vi "WallDistance.vi"(8 "Nominal Angle":dbl=90.0 format="%#_13g", 11 "Points":cluster{"X":sgl, "Y":sgl}[](array[cluster]) {"Y" format="%.2f"; "X" format="%.2f"}) -> (0 "Angle (deg)":dbl, 1 "y-Mean":sgl, 2 "x-Mean":sgl, 3 "Valid":bool, 4 "Segment":T1 {"Point 2"."Y" format="%.2f"; "Point 2"."X" format="%.2f"; "Point 1"."Y" format="%.2f"; "Point 1"."X" format="%.2f"}, 5 "Graph":cluster{sgl[], sgl[]})   [LabVIEW 2015]
uses:
  <vilib>/vision/NI_Vision_Development_Module.lvlib
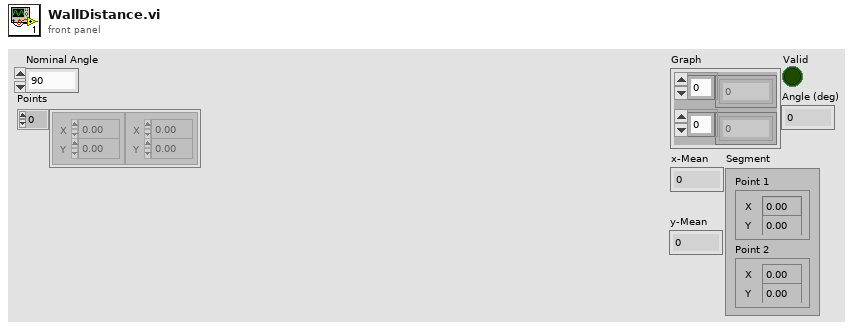
[diagram p1: front panel]
types:
  T1 = cluster{"Point 1":cluster{"X":sgl, "Y":sgl}, "Point 2":cluster{"X":sgl, "Y":sgl}}
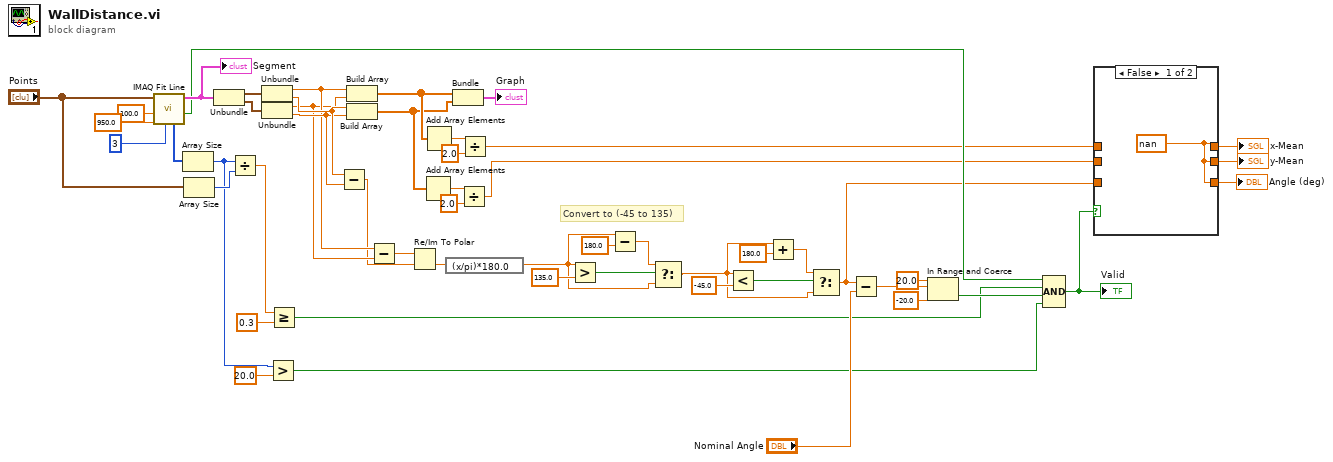
[diagram p0: block diagram]
diagram:
  # "Convert to (-45 to 135)"
  n1 = call "IMAQ Fit Line"("Maximum Iterations"=3, "Pixel Radius"=sgl 100.0, "Minimum Score"=sgl 950.0, "Points"="Points") -> ("Valid Fit?"=w16:bool, "Line Segment"=w21:T1, "Indexes of Points Used"=w23:i32[])  [unwired: 2 in, 3 out]
  "Segment" <- w21
  n2 = Array Size(array=w23) -> (size(s)=w10:i32)
  n3 = Array Size(array="Points") -> (size(s)=w22:i32)
  n4 = Unbundle(w21) -> ("Point 1"=w52:cluster{"X":sgl, "Y":sgl}, "Point 2"=w51:cluster{"X":sgl, "Y":sgl})
  n5 = Divide(x=w10, y=w22) -> (x/y=w15:dbl)
  n6 = Unbundle(w52) -> ("X"=w41:sgl, "Y"=w43:sgl)
  n7 = Unbundle(w51) -> ("X"=w40:sgl, "Y"=w42:sgl)
  n8 = Greater?(x=w10, y=20.0) -> (0:w9:bool)
  n9 = Greater Or Equal?(x=w15, y=0.3) -> (x >= y?=w13:bool)
  n10 = Subtract(x=w43, y=w42) -> (x-y=w38:sgl)
  n11 = Build Array(w41, w40) -> (w49:sgl[])
  n12 = Build Array(w43, w42) -> (w44:sgl[])
  n13 = Subtract(x=w41, y=w40) -> (x-y=w39:sgl)
  n14 = Re/Im To Polar(2:w38, 3:w39) -> (0:w28:sgl)  [unwired: 1 out]
  n15 = Add Array Elements(numeric array=w44) -> (sum=w45:sgl)
  n16 = Add Array Elements(numeric array=w49) -> (sum=w48:sgl)
  n17 = expression code="(x/pi)*180.0" ("radians to degrees")(w28) -> (w27:sgl)
  n18 = Bundle(w49, w44) -> (→"Graph":cluster{sgl[], sgl[]})  [unwired: 1 in]
  n19 = Divide(x=w45, y=sgl 2.0) -> (x/y=w5:sgl)
  n20 = Divide(x=w48, y=sgl 2.0) -> (x/y=w4:sgl)
  n21 = Greater?(x=w27, y=135.0) -> (0:w35:bool)
  n22 = Subtract(x=w27, y=180.0) -> (x-y=w34:dbl)
  n23 = Select(t=w34, s=w35, f=w27) -> (s? t:f=w29:dbl)
  n24 = Less?(x=w29, y=-45.0) -> (x < y?=w32:bool)
  n25 = Add(x=w29, y=180.0) -> (x+y=w33:dbl)
  n26 = Select(t=w33, s=w32, f=w29) -> (s? t:f=w8:dbl)
  n27 = Subtract(x=w8, y="Nominal Angle") -> (x-y=w18:dbl)
  n28 = In Range and Coerce(upper limit=20.0, x=w18, lower limit=-20.0) -> (In Range?=w17:bool)  [unwired: 1 out]
  n29 = Compound Arithmetic op=AND(w16, w13, w17, w9) -> (w2:bool)
  "Valid" <- w2
  n30 = case shown="False" w2 {
    tunnel: w8 -> [_ w56]
    tunnel: [w53 w56] -> w7
    tunnel: [w53 w55] -> w6
    tunnel: w5 -> [_ w55]
    tunnel: w4 -> [_ w54]
    tunnel: [w53 w54] -> w3
    frame False {
      w53 = sgl nan
    }
    frame True {
    }
  }
  "x-Mean" <- w3
  "y-Mean" <- w6
  "Angle (deg)" <- w7
